vi "BoilerRoom AlarmGraph.vi"() -> ()   [LabVIEW 2023]
uses:
  Heater.vi
  AC.vi
panel:
  out "Waveform Chart":i32(graph)
  out "Message":string
  out "Alarm":bool
  out "temp":dbl
  in  "?":dbl(knob) min=0.0 max=2.0 step=1.0 scale=0.0..2.0
  in  "stop":bool
  out "Thermometer":dbl(slide) scale=0.0..100.0
  in  "min temp":dbl=20.0
  in  "max temp":dbl=80.0
  in  "Automatic / Manual":bool
  out "AC":bool
  out "Heater":bool
  # "Heater"
  # "OFF"
  # "AC"
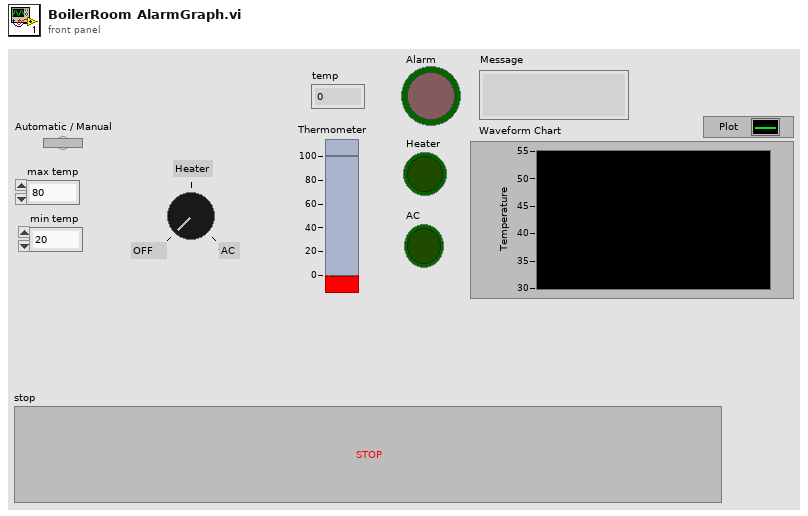
[diagram p1: front panel]
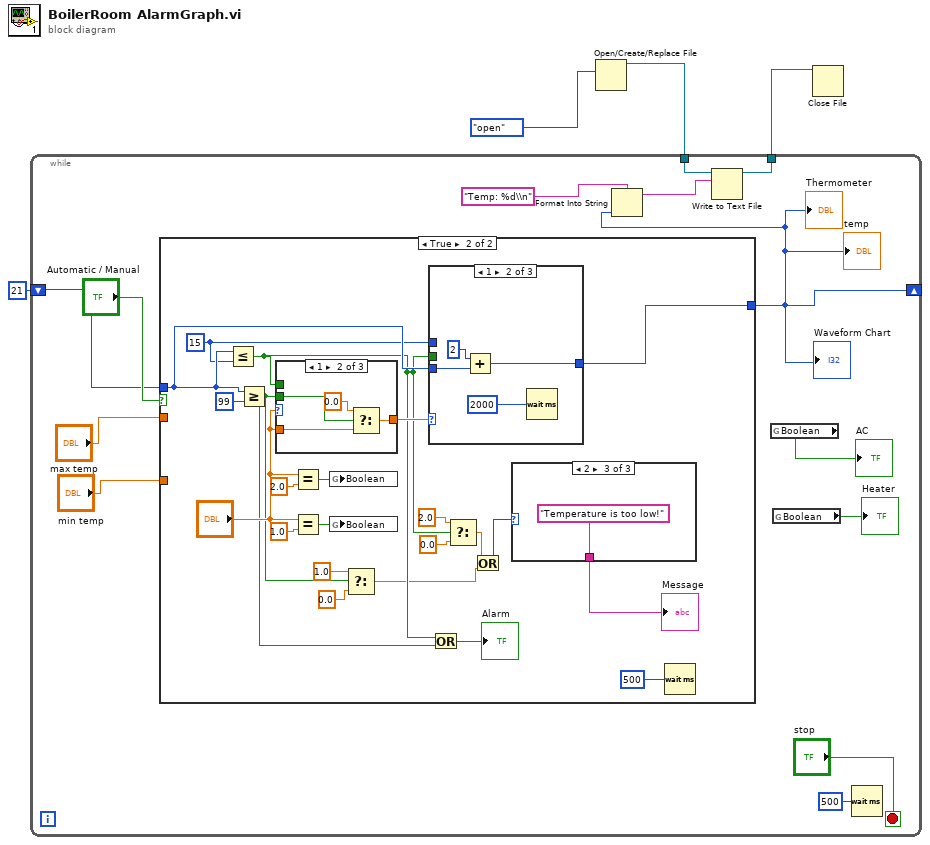
[diagram p0: block diagram]
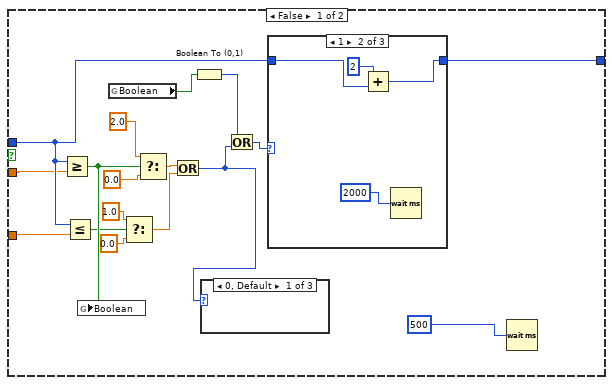
[diagram p2: hidden frame]
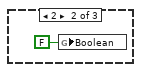
[diagram p3: hidden frame]
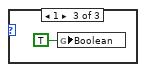
[diagram p4: hidden frame]
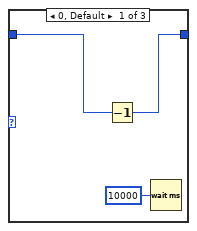
[diagram p5: hidden frame]
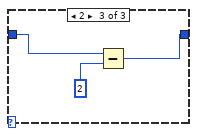
[diagram p6: hidden frame]
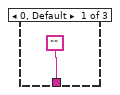
[diagram p7: hidden frame]
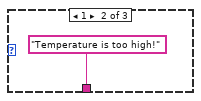
[diagram p8: hidden frame]
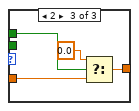
[diagram p10: hidden frame]
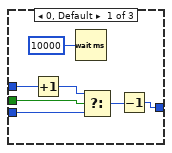
[diagram p11: hidden frame]
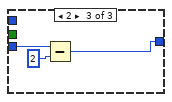
[diagram p12: hidden frame]
diagram:
  n1 = Open/Create/Replace File(operation (0:open)=enum16{"open", "replace"}."open") -> (refnum out=w2:refnum<file>)  [unwired: 5 in, 2 out]
  n2 = while {
    shift-right: [w6] -> _
    shift-left: 21 -> [w10]
    tunnel: w2 -> [w9]
    tunnel: [w8] -> w1
    stop <- "stop" stop-if-true
    n3 = case shown="True" "Automatic / Manual" {
      tunnel: w10 -> [w27 w61]
      tunnel: "max temp" -> [w26 _]
      tunnel: "min temp" -> [w25 _]
      tunnel: [w29 w67] -> w6
      frame False {
        n4 = Greater Or Equal?(x=w27, y=w26) -> (x >= y?=w23:bool)
        n5 = Less Or Equal?(x=w27, y=w25) -> (x <= y?=w22:bool)
        n6 = global write "AC.vi" "Boolean"(w23) -> ()
        n7 = global read "Heater.vi" "Boolean"() -> (w18:bool)
        n8 = Select(t=1.0, s=w22, f=0.0) -> (s? t:f=w24:dbl)
        n9 = Select(t=2.0, s=w23, f=0.0) -> (s? t:f=w30:dbl)
        n10 = Or(x=w30, y=w24) -> (x .or. y?=w21:i32)
        n11 = Boolean To (0,1)(Boolean=w18) -> (0, 1=w19:i16)
        n12 = case shown="0, Default" w21 {
          frame 0, Default {
          }
          frame 2 {
            n13 = global write "Heater.vi" "Boolean"(FALSE ("Boolean")) -> ()
          }
          frame 1 {
            n14 = global write "Heater.vi" "Boolean"(TRUE ("Boolean")) -> ()
          }
        }
        n15 = Or(x=w19, y=w21) -> (x .or. y?=w20:i32)
        n16 = case shown="1" w20 {
          tunnel: w27 -> [w39 w43 w46]
          tunnel: [w38 w41 w45] -> w29
          frame 0, Default {
            n17 = Decrement(x=w39) -> (x-1=w38:i32)
            n18 = Wait (ms)(milliseconds to wait=u32 10000) -> ()  [unwired: 1 out]
          }
          frame 1 {
            n19 = Add(x=2, y=w43) -> (x+y=w41:i32)
            n20 = Wait (ms)(milliseconds to wait=u32 2000) -> ()  [unwired: 1 out]
          }
          frame 2 {
            n21 = Subtract(x=w46, y=2) -> (x-y=w45:i32)
          }
        }
        n22 = Wait (ms)(milliseconds to wait=u32 500) -> ()  [unwired: 1 out]
      }
      frame True {
        w58 = 15
        n23 = Less Or Equal?(x=w61, y=w58) -> (x <= y?=w53:bool)
        n24 = Greater Or Equal?(x=w61, y=99 ("x")) -> (x >= y?=w52:bool)
        n25 = case shown="1" "?" {
          tunnel: "?" -> [w72 w73 w78]
          tunnel: [w72 w75 w79] -> w66
          tunnel: w52 -> [_ w76 _]
          tunnel: w53 -> [_ _ w80]
          frame 0, Default {
          }
          frame 1 {
            n26 = Select(t=0.0 ("f"), s=w76, f=w73) -> (s? t:f=w75:dbl)
          }
          frame 2 {
            n27 = Select(t=0.0, s=w80, f=w78) -> (s? t:f=w79:dbl)
          }
        }
        n28 = Equal?(x="?", y=2.0) -> (x = y?=w62:bool)
        n29 = Equal?(x="?", y=1.0) -> (x = y?=w64:bool)
        n30 = global write "AC.vi" "Boolean"(w62) -> ()
        n31 = global write "Heater.vi" "Boolean"(w64) -> ()
        n32 = Select(t=1.0, s=w52, f=0.0) -> (s? t:f=w49:dbl)
        n33 = case shown="1" w66 {
          tunnel: w61 -> [w84 w91 w94]
          tunnel: [w87 w90 w93] -> w67
          tunnel: w53 -> [w85 _ _]
          tunnel: w58 -> [w82 _ _]
          frame 0, Default {
            n34 = Increment(x=w82) -> (x+1=w81:i32)
            n35 = Wait (ms)(milliseconds to wait=u32 10000) -> ()  [unwired: 1 out]
            n36 = Select(t=w81, s=w85, f=w84) -> (s? t:f=w83:i32)
            n37 = Decrement(x=w83) -> (x-1=w87:i32)
          }
          frame 1 {
            n38 = Add(x=2, y=w91) -> (x+y=w90:i32)
            n39 = Wait (ms)(milliseconds to wait=u32 2000) -> ()  [unwired: 1 out]
          }
          frame 2 {
            n40 = Subtract(x=w94, y=2) -> (x-y=w93:i32)
          }
        }
        n41 = Or(x=w53, y=w52) -> (x .or. y?=→"Alarm":bool)
        n42 = Select(t=2.0, s=w53, f=0.0) -> (s? t:f=w48:dbl)
        n43 = Or(x=w48, y=w49) -> (x .or. y?=w47:i32)
        n44 = case shown="2" w47 {
          tunnel: ["" "Temperature is too high!" "Temperature is too low!"] -> w51
          frame 0, Default {
          }
          frame 1 {
          }
          frame 2 {
          }
        }
        "Message" <- w51
        n45 = Wait (ms)(milliseconds to wait=u32 500) -> ()  [unwired: 1 out]
      }
    }
    "Thermometer" <- w6
    "temp" <- w6
    "Waveform Chart" <- w6
    n46 = Format Into String(format string="Temp: %d\\n", w6) -> (resulting string=w5:string)  [unwired: 2 in, 1 out]
    n47 = Write to Text File(file (use dialog)=w9, text=w5) -> (refnum out=w8:refnum<file>)  [unwired: 2 in, 2 out]
    n48 = global read "AC.vi" "Boolean"() -> (→"AC":bool)
    n49 = global read "Heater.vi" "Boolean"() -> (→"Heater":bool)
    n50 = Wait (ms)(milliseconds to wait=u32 500) -> ()  [unwired: 1 out]
  }
  n51 = Close File(refnum=w1) -> ()  [unwired: 1 in, 2 out]
